vi "packageTelemetrySnapshot.vi"(8 "Error In":errorcluster, 10 "All Data":T1 {"Power Readings"."Current" format="%#.3g A"; "Power Readings"."Power" format="%#.3g W"; "Power Readings"."Shunt Voltage" format=" %#.3g V"; "Power Readings"."Bus Voltage" format="%#.3g V"; "Power Readings"."Voltage (Total)" format="%#.3g V"; "ThermalReadings"."Ambient Temp (°F)" format="%.2f °F"; "ThermalReadings"."Ambient Temp (°C)" format="%.2f °C"; "ThermalReadings"."Object Temp (°F)" format="%.2f °F"; "ThermalReadings"."Object Temp (°C)" format="%.2f °C"; "CPU loads"."ISR (%)" format="%#.2f"; "CPU loads"."Idle (%)" format="%#.2f"; "CPU loads"."Background (%)" format="%#.2f"; "CPU loads"."Normal (%)" format="%#.2f"; "CPU loads"."Above Normal (%)" format="%#.2f"; "CPU loads"."High (%)" format="%#.2f"; "CPU loads"."Timed Structures (%)" format="%#.2f"; "CPU loads"."Time Critical (%)" format="%#.2f"; "CPU loads"."Total (%)" format="%#.2f"}, 11 "Send Non-Critical Data":bool) -> (0 "Error Out":errorcluster, 3 "Latest Critical Telemetry":T10)   [LabVIEW 2014]
uses:
  Type Defs/criticalTelemetry.ctl
  Type Defs/PodState.ctl
  Type Defs/allData.ctl
  Sensors/Power Sensor - Adafruit INA219/INA219 Measurements.ctl
  Type Defs/tempReadings.ctl
  Type Defs/AnalogPressureReading.ctl
  Type Defs/laserReading.ctl
  Type Defs/tofReading.ctl
  <vilib>/Utility/RT CPU Load.ctl
  Type Defs/pressureReading.ctl
  <vilib>/NI_Real-Time Target Support.lvlib
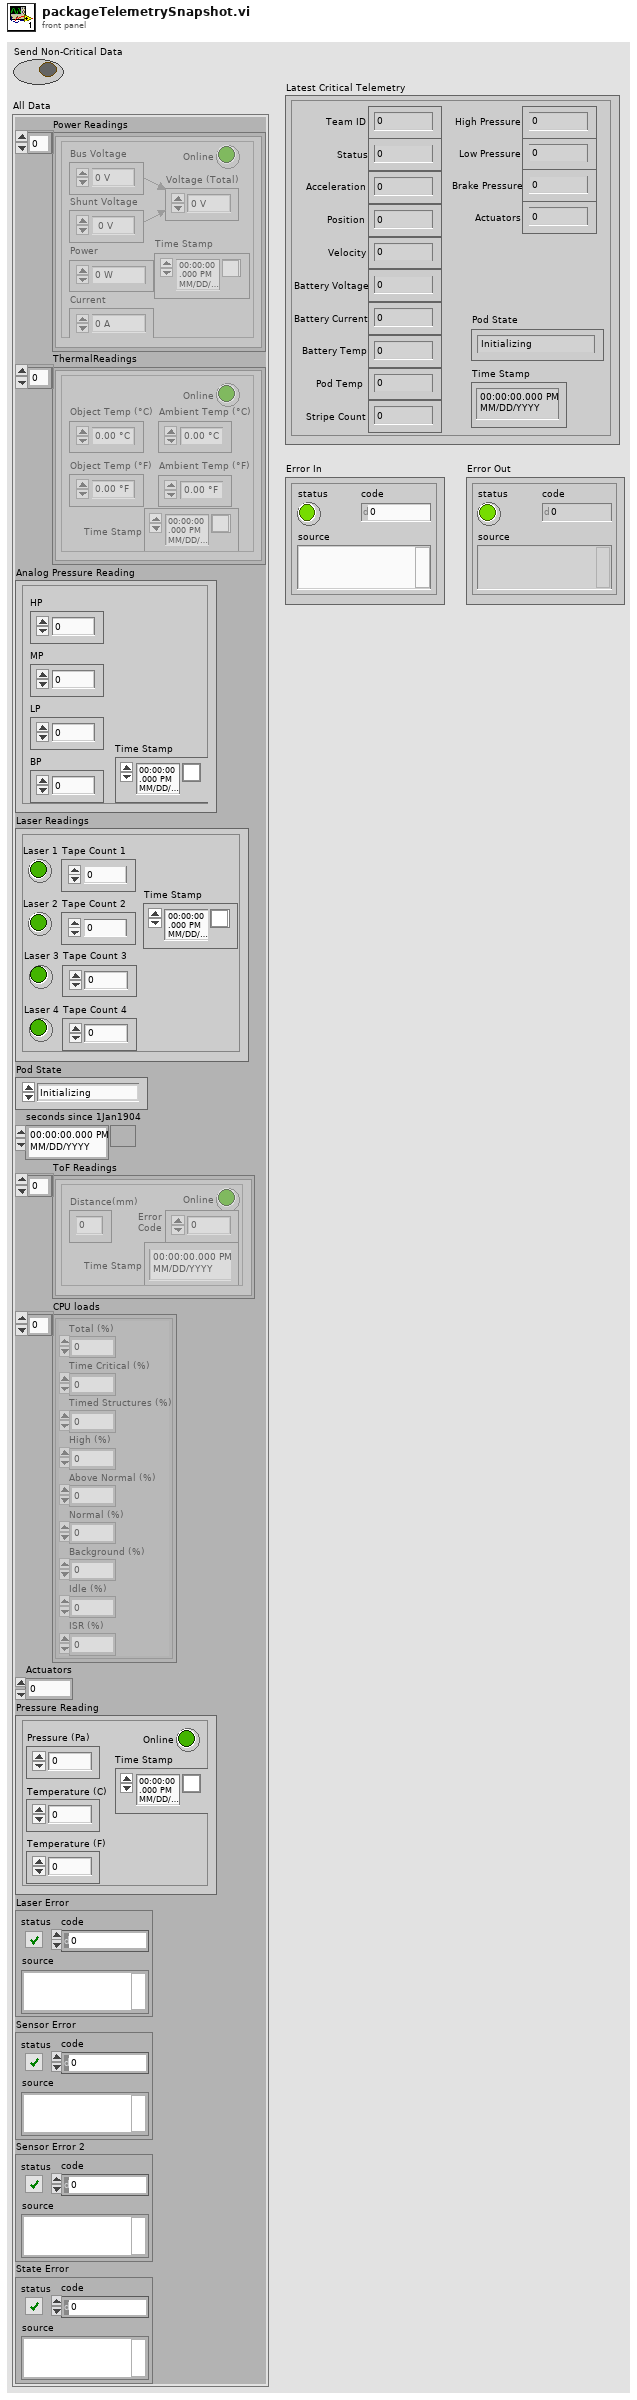
[diagram p1: front panel]
types:
  T1 = typedef "allData.ctl" = cluster{"Power Readings":T2[], "ThermalReadings":T3[], "Analog Pressure Reading":T4, "Laser Readings":T5, "Pod State":T6, "seconds since 1Jan1904":timestamp, "ToF Readings":T7[], "CPU loads":T8[], "Actuators":u32, "Pressure Reading":T9, "Laser Error":errorcluster, "Sensor Error":errorcluster, "Sensor Error 2":errorcluster, "State Error":errorcluster}
  T2 = typedef "INA219 Measurements.ctl" = cluster{"Voltage (Total)":dbl, "Bus Voltage":dbl, "Shunt Voltage":dbl, "Power":dbl, "Current":dbl, "Online":bool, "Time Stamp":timestamp}
  T3 = typedef "tempReadings.ctl" = cluster{"Object Temp (°C)":dbl, "Object Temp (°F)":dbl, "Ambient Temp (°C)":dbl, "Ambient Temp (°F)":dbl, "Online":bool, "Time Stamp":timestamp}
  T4 = typedef "AnalogPressureReading.ctl" = cluster{"HP":dbl, "MP":dbl, "LP":dbl, "BP":dbl, "Time Stamp":timestamp}
  T5 = typedef "laserReading.ctl" = cluster{"Laser 1":bool, "Tape Count 1":u32, "Laser 2":bool, "Tape Count 2":u32, "Laser 3":bool, "Tape Count 3":u32, "Laser 4":bool, "Tape Count 4":u32, "Time Stamp":timestamp}
  T6 = typedef "PodState.ctl" = enum16{"Initializing", "Pre-flight Testing", "Ready", "Pushing", "Coast", "Braking", "Post-flight", "Fault"}
  T7 = typedef "tofReading.ctl" = cluster{"Distance(mm)":u8, "Online":bool, "Error\nCode":u8, "Time Stamp":timestamp}
  T8 = typedef "NI_Real-Time Target Support.lvlib/RT CPU Load.ctl" = cluster{"Total (%)":dbl, "Time Critical (%)":dbl, "Timed Structures (%)":dbl, "High (%)":dbl, "Above Normal (%)":dbl, "Normal (%)":dbl, "Background (%)":dbl, "Idle (%)":dbl, "ISR (%)":dbl}
  T9 = typedef "pressureReading.ctl" = cluster{"Time Stamp":timestamp, "Online":bool, "Temperature (C)":dbl, "Pressure (Pa)":dbl, "Temperature (F)":dbl}
  T10 = typedef "criticalTelemetry.ctl" = cluster{"Team ID":u8, "Status":u8, "Acceleration":i32, "Position":i32, "Velocity":i32, "Battery Voltage":i32, "Battery Current":i32, "Battery Temp":i32, "Pod Temp":i32, "Stripe Count":u32, "High Pressure":dbl, "Low Pressure":dbl, "Brake Pressure":dbl, "Actuators":u32, "Pod State":T6, "Time Stamp":timestamp}
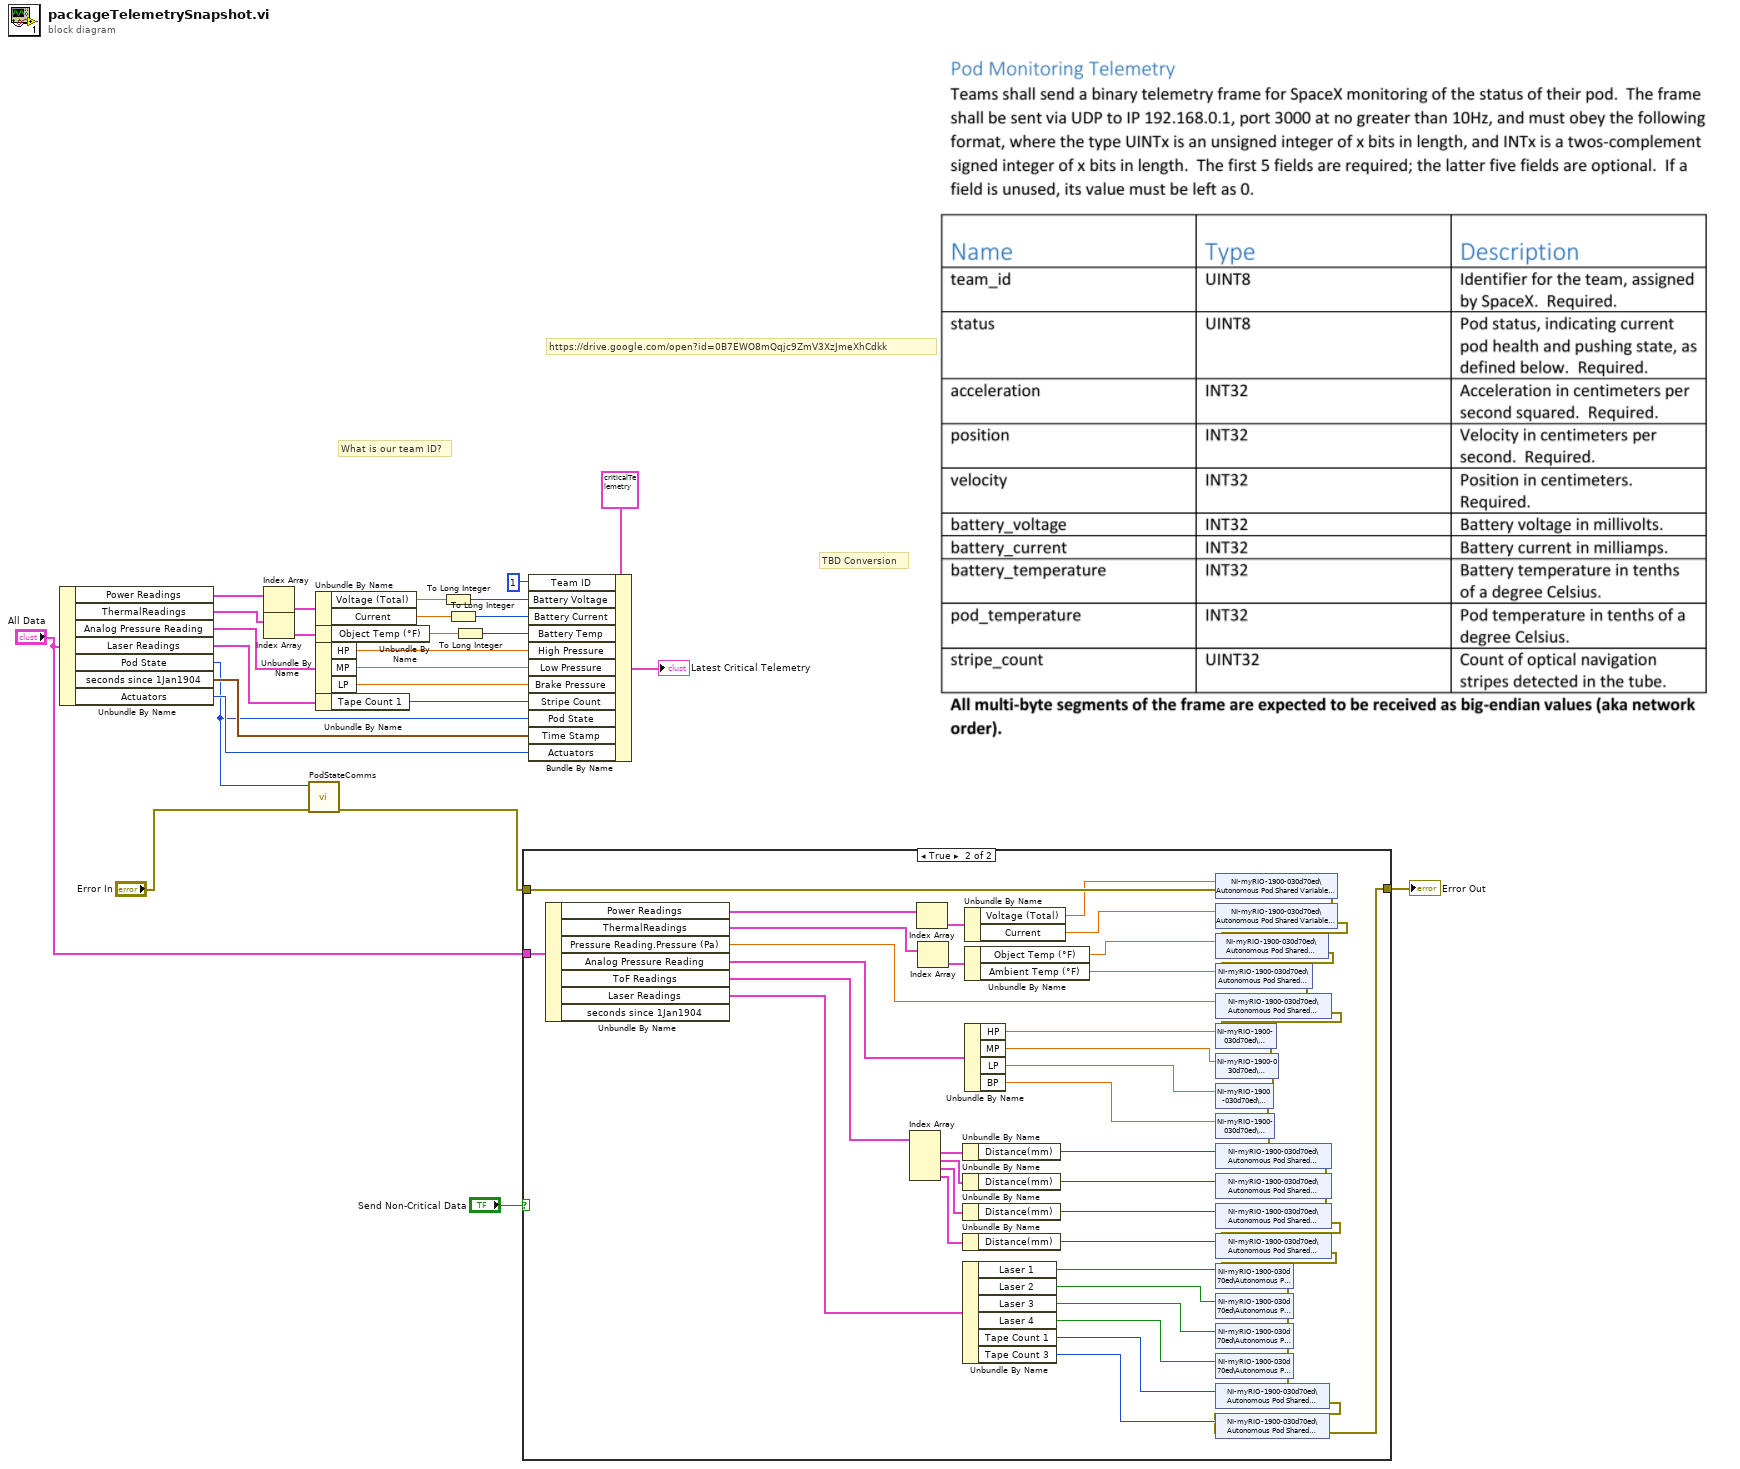
[diagram p0: block diagram]
diagram:
  # "What is our team ID?"
  # "https://drive.google.com/open?id=0B7EWO8mQqjc9ZmV3XzJmeXhCdkk"
  # "TBD Conversion"
  n1 = Unbundle By Name("All Data") -> ("Power Readings"=w27:T2[], "ThermalReadings"=w22:T3[], "Analog Pressure Reading"=w19:T4, "Laser Readings"=w15:T5, "Pod State"=w3:T6, "seconds since 1Jan1904"=w14:timestamp, "Actuators"=w4:u32)
  n2 = Index Array(array=w27) -> (element=w25:T2)  [unwired: 1 in]
  n3 = Index Array(array=w22) -> (element=w21:T3)  [unwired: 1 in]
  n4 = call "PodStateComms.vi"("error in"="Error In", "Pod State"=w3) -> ("error out"=w1:errorcluster)  [unwired: 9 in]
  n5 = Unbundle By Name(w25) -> ("Voltage (Total)"=w24:dbl, "Current"=w23:dbl)
  n6 = Unbundle By Name(w21) -> ("Object Temp (°F)"=w20:dbl)
  n7 = Unbundle By Name(w19) -> ("HP"=w18:dbl, "MP"=w17:dbl, "LP"=w16:dbl)
  n8 = Unbundle By Name(w15) -> ("Tape Count 1"=w11:u32)
  n9 = To Long Integer(number=w24) -> (32bit integer=w10:i32)
  n10 = To Long Integer(number=w23) -> (32bit integer=w9:i32)
  n11 = To Long Integer(number=w20) -> (32bit integer=w8:i32)
  n12 = case shown="True" "Send Non-Critical Data" {
    tunnel: "All Data" -> [_ w74]
    tunnel: w1 -> [w28 w73]
    tunnel: [w28 w29] -> w5
    frame False {
    }
    frame True {
      n13 = Unbundle By Name(w74) -> ("Power Readings"=w75:T2[], "ThermalReadings"=w77:T3[], "Pressure Reading.Pressure (Pa)"=w68:dbl, "Analog Pressure Reading"=w79:T4, "ToF Readings"=w63:T7[], "Laser Readings"=w54:T5)  [unwired: 1 out]
      n14 = Index Array(array=w63) -> (element #1=w62:T7, element #2=w55:T7, element #3=w56:T7, element #4=w57:T7)  [unwired: 4 in]
      n15 = Index Array(array=w75) -> (element=w76:T2)  [unwired: 1 in]
      n16 = Index Array(array=w77) -> (element=w78:T3)  [unwired: 1 in]
      n17 = Unbundle By Name(w62) -> ("Distance(mm)"=w61:u8)
      n18 = Unbundle By Name(w55) -> ("Distance(mm)"=w58:u8)
      n19 = Unbundle By Name(w56) -> ("Distance(mm)"=w59:u8)
      n20 = Unbundle By Name(w57) -> ("Distance(mm)"=w60:u8)
      n21 = Unbundle By Name(w54) -> ("Laser 1"=w53:bool, "Laser 2"=w52:bool, "Laser 3"=w51:bool, "Laser 4"=w50:bool, "Tape Count 1"=w49:u32, "Tape Count 3"=w48:u32)
      n22 = Unbundle By Name(w76) -> ("Voltage (Total)"=w72:dbl, "Current"=w71:dbl)
      n23 = Unbundle By Name(w78) -> ("Object Temp (°F)"=w70:dbl, "Ambient Temp (°F)"=w69:dbl)
      n24 = Unbundle By Name(w79) -> ("HP"=w67:dbl, "MP"=w66:dbl, "LP"=w65:dbl, "BP"=w64:dbl)
      n25 = shared-variable "NI-myRIO-1900-030d70ed\\Autonomous Pod Shared Variables.lvlib\\BatteryVoltage"(w72, error in=w73) -> (error out=w47:errorcluster)
      n26 = shared-variable "NI-myRIO-1900-030d70ed\\Autonomous Pod Shared Variables.lvlib\\BatteryCurrent"(w71, error in=w47) -> (error out=w46:errorcluster)
      n27 = shared-variable "NI-myRIO-1900-030d70ed\\Autonomous Pod Shared Variables.lvlib\\BatteryTemp"(w70, error in=w46) -> (error out=w45:errorcluster)
      n28 = shared-variable "NI-myRIO-1900-030d70ed\\Autonomous Pod Shared Variables.lvlib\\PodTemp"(w69, error in=w45) -> (error out=w44:errorcluster)
      n29 = shared-variable "NI-myRIO-1900-030d70ed\\Autonomous Pod Shared Variables.lvlib\\TubePressure"(w68, error in=w44) -> (error out=w43:errorcluster)
      n30 = shared-variable "NI-myRIO-1900-030d70ed\\Autonomous Pod Shared Variables.lvlib\\HP"(w67, error in=w43) -> (error out=w42:errorcluster)
      n31 = shared-variable "NI-myRIO-1900-030d70ed\\Autonomous Pod Shared Variables.lvlib\\MP"(w66, error in=w42) -> (error out=w41:errorcluster)
      n32 = shared-variable "NI-myRIO-1900-030d70ed\\Autonomous Pod Shared Variables.lvlib\\LP"(w65, error in=w41) -> (error out=w40:errorcluster)
      n33 = shared-variable "NI-myRIO-1900-030d70ed\\Autonomous Pod Shared Variables.lvlib\\BP"(w64, error in=w40) -> (error out=w39:errorcluster)
      n34 = shared-variable "NI-myRIO-1900-030d70ed\\Autonomous Pod Shared Variables.lvlib\\ToF1Distance"(w61, error in=w39) -> (error out=w38:errorcluster)
      n35 = shared-variable "NI-myRIO-1900-030d70ed\\Autonomous Pod Shared Variables.lvlib\\ToF2Distance"(w58, error in=w38) -> (error out=w37:errorcluster)
      n36 = shared-variable "NI-myRIO-1900-030d70ed\\Autonomous Pod Shared Variables.lvlib\\ToF3Distance"(w59, error in=w37) -> (error out=w36:errorcluster)
      n37 = shared-variable "NI-myRIO-1900-030d70ed\\Autonomous Pod Shared Variables.lvlib\\ToF4Distance"(w60, error in=w36) -> (error out=w35:errorcluster)
      n38 = shared-variable "NI-myRIO-1900-030d70ed\\Autonomous Pod Shared Variables.lvlib\\Laser1"(w53, error in=w35) -> (error out=w34:errorcluster)
      n39 = shared-variable "NI-myRIO-1900-030d70ed\\Autonomous Pod Shared Variables.lvlib\\Laser2"(w52, error in=w34) -> (error out=w33:errorcluster)
      n40 = shared-variable "NI-myRIO-1900-030d70ed\\Autonomous Pod Shared Variables.lvlib\\Laser3"(w51, error in=w33) -> (error out=w32:errorcluster)
      n41 = shared-variable "NI-myRIO-1900-030d70ed\\Autonomous Pod Shared Variables.lvlib\\Laser4"(w50, error in=w32) -> (error out=w31:errorcluster)
      n42 = shared-variable "NI-myRIO-1900-030d70ed\\Autonomous Pod Shared Variables.lvlib\\StripeCount1"(w49, error in=w31) -> (error out=w30:errorcluster)
      n43 = shared-variable "NI-myRIO-1900-030d70ed\\Autonomous Pod Shared Variables.lvlib\\StripeCount2"(w48, error in=w30) -> (error out=w29:errorcluster)
    }
  }
  "Error Out" <- w5
  n44 = Bundle By Name(cluster=T10 {"Team ID"=0, "Status"=0, "Acceleration"=0, "Position"=0, "Velocity"=0, "Battery Voltage"=0, "Battery Current"=0, "Battery Temp"=0, "Pod Temp"=0, "Stripe Count"=0, "High Pressure"=0.0, "Low Pressure"=0.0, "Brake Pressure"=0.0, "Actuators"=0, "Pod State"=enum."Initializing", "Time Stamp"=timestamp(0 s since 1904-01-01)} ("Latest Critical Telemetry"), "Team ID"=u8 1, "Battery Voltage"=w10, "Battery Current"=w9, "Battery Temp"=w8, "High Pressure"=w18, "Low Pressure"=w17, "Brake Pressure"=w16, "Stripe Count"=w11, "Pod State"=w3, "Time Stamp"=w14, "Actuators"=w4) -> (→"Latest Critical Telemetry":T10)
